vi "TAI_Servo.vi"(3 "Normal Output":dbl, 4 "Override Actuator Bypass":bool, 5 "Actuator Name":string) -> (0 "Interlocked Output":dbl, 2 "Output Mode":T1(ring))   [LabVIEW 2020]
doc: "This VI is configured for polymorphic use and functions as an interlock, allowing the selected servo to be tested manually via the FRC 4265 Dashboard. During testing, all interlocked actuators which are not selected for testing are disabled."
uses:
  cf260dee-87cd-4ad6-a0e3-c3116b7c1a2f.vi
  e00df7bd-b999-461d-9362-47e176d3d7d1.vi
  driverdata.vi
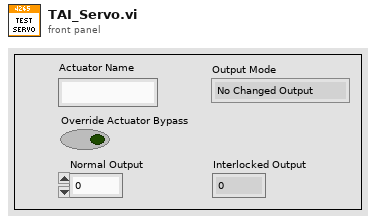
[diagram p1: front panel]
types:
  T1 = enum16{"No Changed Output", "New Normal Output", "New Testing Output"}
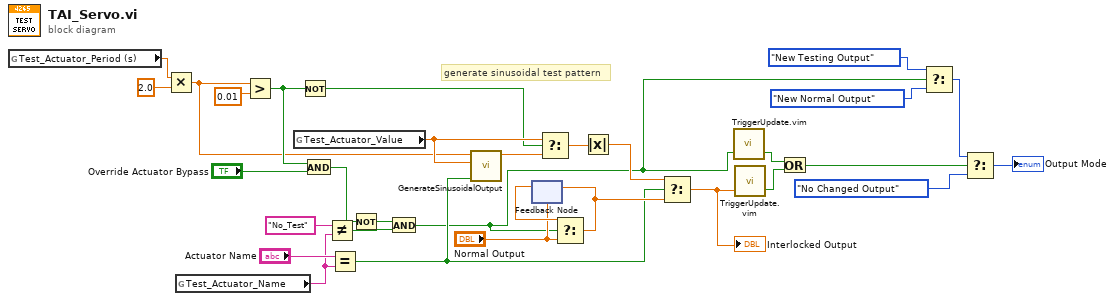
[diagram p0: block diagram]
diagram:
  # "generate sinusoidal test pattern"
  n1 = global read "driverdata.vi" "Test_Actuator_Period (s)"() -> (w14:dbl)
  n2 = Multiply(x=w14, y=2.0) -> (x*y=w13:dbl)
  n3 = global read "driverdata.vi" "Test_Actuator_Name"() -> (w29:string)
  n4 = Greater?(x=w13, y=0.01) -> (0:w17:bool)
  n5 = global read "driverdata.vi" "Test_Actuator_Value"() -> (w24:dbl)
  n6 = Not(x=w17) -> (.not. x?=w12:bool)
  n7 = And(x=w17, y="Override Actuator Bypass") -> (x .and. y?=w20:bool)
  n8 = Not Equal?(x="No_Test", y=w29) -> (x != y?=w18:bool)
  n9 = Equal?(x="Actuator Name", y=w29) -> (x = y?=w2:bool)
  n10 = Not(x=w20) -> (.not. x?=w19:bool)
  n11 = And(x=w19, y=w18) -> (x .and. y?=w1:bool)
  n12 = call "GenerateSinusoidalOutput.vi"("Init"=w2, "Amplitude"=w24, "Period (s)"=w13) -> ("sin(time)"=w25:dbl)  [unwired: 8 in]
  n13 = feedback #1("Normal Output") -> (w28:dbl)
  n14 = Select(t=w24, s=w12, f=w25) -> (s? t:f=w23:dbl)
  n15 = Select(t=w28, s=w1, f="Normal Output") -> (s? t:f=w26:dbl)
  n16 = feedback-in #1(w26) -> ()
  n17 = Absolute Value(x=w23) -> (abs(x)=w16:dbl)
  n18 = Select(t=w16, s=w2, f=w26) -> (s? t:f=w6:dbl)
  "Interlocked Output" <- w6
  n19 = call "TriggerUpdate.vim"("Trigger"=w1) -> ("Update"=w5:bool)  [unwired: 2 in]
  n20 = call "TriggerUpdate.vim"("Trigger"=w6) -> ("Update"=w4:bool)  [unwired: 2 in]
  n21 = Or(x=w5, y=w4) -> (x .or. y?=w3:bool)
  n22 = Select(t=T1."New Testing Output", s=w1, f=T1."New Normal Output") -> (s? t:f=w9:T1)
  n23 = Select(t=w9, s=w3, f=T1."No Changed Output") -> (s? t:f=→"Output Mode":T1)
